vi "Write Analogue.vi"(8 "error in (no error)":errorcluster, 9 "Output":bool, 10 "Channel index(0)":i32, 11 "Keysight 6700C in":refnum<class "Keysight 6700C.lvclass">) -> (0 "error out":errorcluster, 2 "Success?":bool, 3 "Keysight 6700C out":refnum<class "Keysight 6700C.lvclass">)   [LabVIEW 2025, in "Power Supply.lvlib" / "Keysight 6700C.lvclass"]
uses:
  Keysight 6700C.lvclass
  Keysight 6700C.lvclass/Keysight 6700C.ctl
  <instrlib>/Agilent N6700 Series/Agilent N6700 Series.lvlib
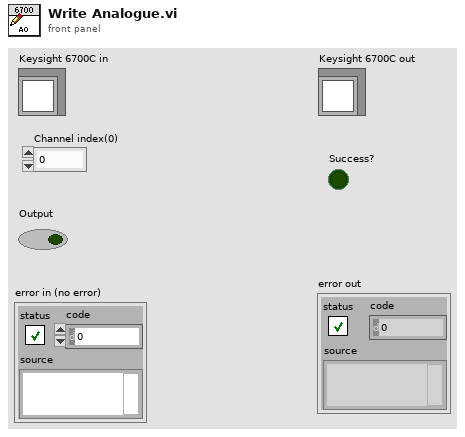
[diagram p1: front panel]
types:
  T1 = typedef "Abstract Engine.lvlibp/Abstract Instrument.lvclass/Channel.ctl" = cluster{"Index":i32, "Alias":string, "Unit":T2, "Upper limit":dbl, "Lower limit":dbl, "Measurement":variant}
  T2 = typedef "Abstract Engine.lvlibp/Abstract Instrument.lvclass/Unit.ctl" = enum16{"V", "A", "Ohm", "Hz", "uF", "degC", "deg"}
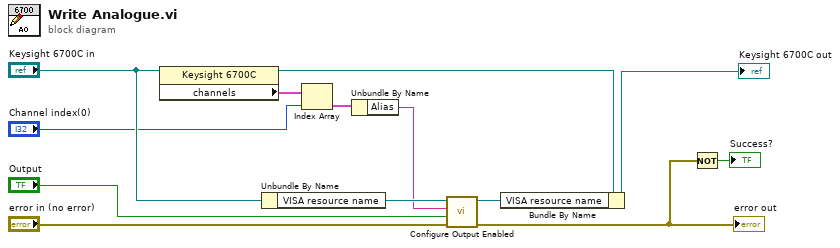
[diagram p0: block diagram]
diagram:
  n1 = property class="Keysight 6700C"(reference="Keysight 6700C in") -> (reference out=w4:refnum<class "Keysight 6700C.lvclass">, "channels"=w3:T1[])  [unwired: 1 in, 1 out]
  n2 = Unbundle By Name("Keysight 6700C in") -> ("VISA resource name"=w12:refnum<visa-resource-name>)
  n3 = Index Array(array=w3, index="Channel index(0)") -> (element=w2:T1)
  n4 = Unbundle By Name(w2) -> ("Alias"=w1:string)
  n5 = call <instrlib>:"Configure Output Enabled.vi"("error in (no error)"="error in (no error)", "Enable Output (False)"="Output", "Channel Name (1)"=w1, "VISA resource name"=w12) -> ("error out"=w9:errorcluster, "VISA resource name out"=w5:refnum<visa-resource-name>)  [unwired: 6 in]
  "error out" <- w9
  n6 = Bundle By Name(cluster=w4, "VISA resource name"=w5) -> (→"Keysight 6700C out":refnum<class "Keysight 6700C.lvclass">)
  n7 = Not(x=w9) -> (.not. x?=→"Success?":bool)
